vi "count_run 1.vi"(7 "cmd":T1, 8 "error in (no error)":errorcluster, 9 "CH":i32, 11 "Array_Count":dbl[](array[numeric])) -> (0 "error out":errorcluster, 3 "Array_data":dbl[][](array[numeric]))   [LabVIEW 2019]
uses:
  cmd_count.ctl
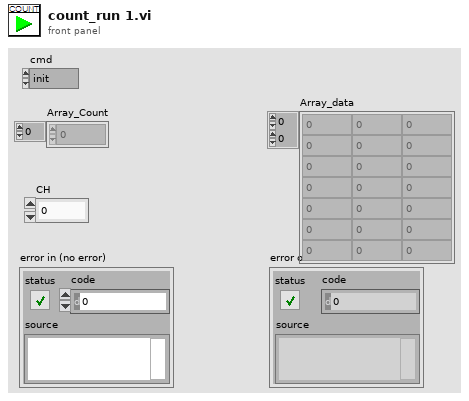
[diagram p1: front panel]
types:
  T1 = typedef "cmd_count.ctl" = enum16{"init", "count", "default"}
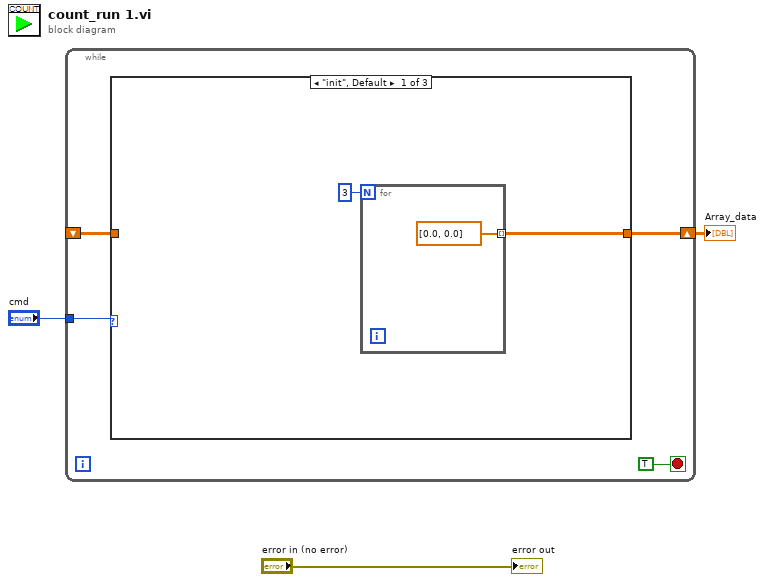
[diagram p0: block diagram]
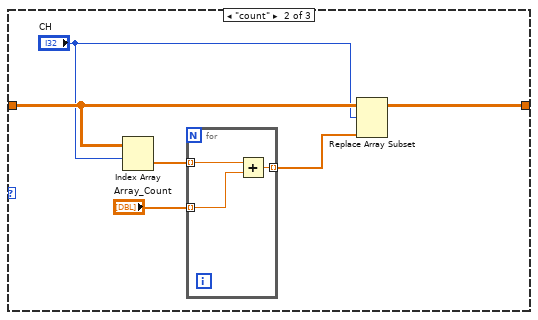
[diagram p2: hidden frame]
diagram:
  n1 = while {
    tunnel: "cmd" -> [w6]
    shift-right: [w5] -> w1
    shift-left: _ -> [w4]
    stop <- TRUE stop-if-true
    n2 = case shown="\"init\", Default" w6 {
      tunnel: [w8 w11 w20] -> w5
      tunnel: w4 -> [_ w16 w20]
      frame "init", Default {
        n3 = for {
          N: 3 -> [_]
          tunnel: [dbl[] [0.0, 0.0]] -> w8 mode=indexing
        }
      }
      frame "count" {
        n4 = Index Array(array=w16, index (row)="CH") -> (element=w14:dbl[])  [unwired: 1 in]
        n5 = for {
          tunnel: w14 -> [w19] mode=indexing
          tunnel: "Array_Count" -> [w18] mode=indexing
          tunnel: [w17] -> w12 mode=indexing
          n6 = Add(x=w19, y=w18) -> (x+y=w17:dbl)
        }
        n7 = Replace Array Subset(array=w16, new element=w12, index (row)="CH") -> (w11:dbl[][])  [unwired: 1 in]
      }
      frame "default" {
      }
    }
  }
  "Array_data" <- w1
  "error out" <- "error in (no error)"
